vi "MyInterfaceMethod.vi"(0 "reference in":refnum<class "IMyInterface2.lvclass">, 1 "MyParameter":dbl, 5 "error in (no error)":errorcluster) -> (14 "reference out":refnum<class "IMyInterface2.lvclass">, 19 "error out":errorcluster)   [LabVIEW 2020, in "IMyInterface2.lvclass"]
uses:
  IMyInterface2.lvclass
  C:/Program Files (x86)/National Instruments/LabVIEW 2020/vi.lib/addons/_AddQ/G#Interface/G#Interface.lvclass
  vi.lib/addons/_AddQ/G#Interface/G#Interface.lvclass
panel:
  # "Only add controls and indicators\nand wire them to the connector pane.\n\nPlease be aware that this VI will execute\nthe implementing method VI by using\nVI server, causing the VI to run top-level.\n\nMake sure that the frontpanel is available\nand never removed from the implementing\nmethod VI . Trick: Just put a reference to\nthe \"reference in\" class control (just as the\nerror case in this VI). This will prevent that\nfrontpanel is removed by LabVIEW."
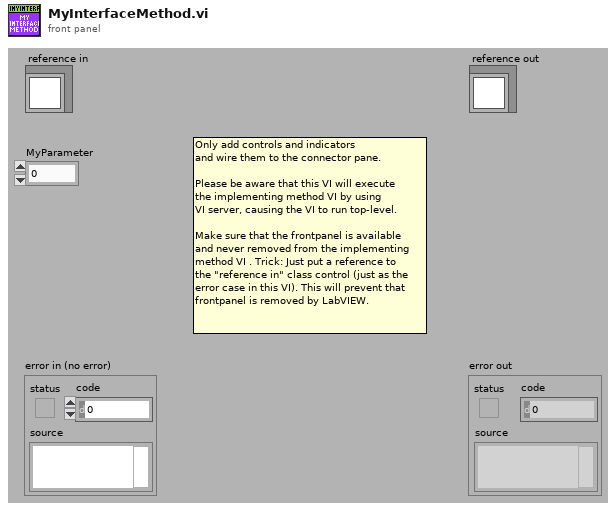
[diagram p1: front panel]
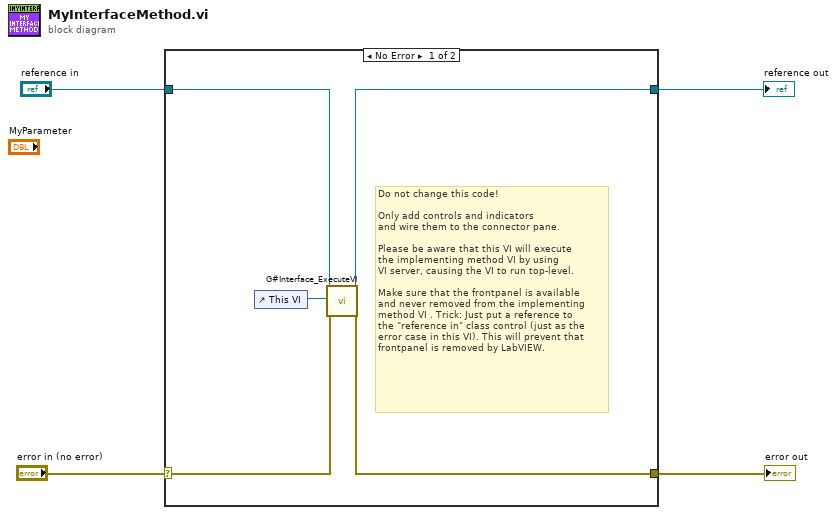
[diagram p0: block diagram]
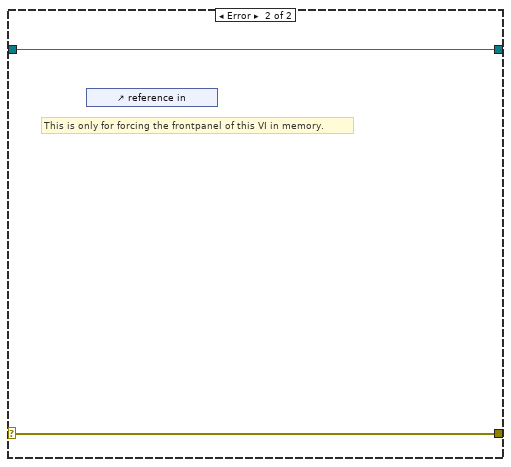
[diagram p2: hidden frame]
diagram:
  n1 = case shown="No Error" "error in (no error)" {
    selector: "error in (no error)" -> [w8 w11]
    tunnel: [w7 w11] -> w3
    tunnel: [w6 w10] -> w1
    tunnel: "reference in" -> [w9 w10]
    frame No Error {
      # "Do not change this code!\n\nOnly add controls and indicators\nand wire them to the connector pane.\n\nPlease be aware that this VI will execute\nthe implementing method VI by using\nVI server, causing the VI to run top-level.\n\nMake sure that the frontpanel is available\nand never removed from the implementing\nmethod VI . Trick: Just put a reference to\nthe \"reference in\" class control (just as the\nerror case in this VI). This will prevent that\nfrontpanel is removed by LabVIEW."
      n2 = control-ref of="This VI"() -> (w5:refnum<vi>)
      n3 = call "G#Interface_ExecuteVI.vi"("reference in"=w9, "VI Refnum"=w5, "error in (no error)"=w8) -> ("reference out"=w6:refnum<class "IMyInterface2.lvclass">, "error out"=w7:errorcluster)  [unwired: 15 in]
    }
    frame Error {
      # "This is only for forcing the frontpanel of this VI in memory."
      n4 = control-ref of="reference in"() -> ()  [unwired: 1 out]
    }
  }
  "error out" <- w3
  "reference out" <- w1
